vi "StringToNumber.vi"(7 "Conversion type":enum16{"float", "dbl"}(ring), 8 "error in":errorcluster, 10 "String array":string[](array[string]), 11 "String":string) -> (0 "error out":errorcluster, 2 "Number array":dbl[](array[numeric]), 3 "Number":dbl)   [LabVIEW 2019, in "Tools.lvlib"]
uses:
  Tools.lvlib
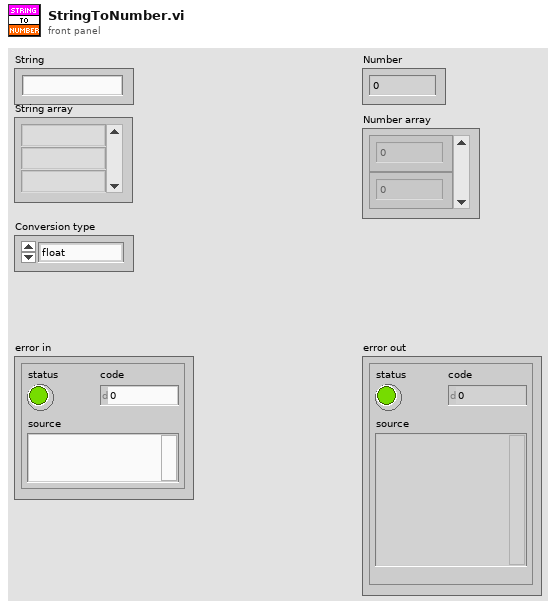
[diagram p1: front panel]
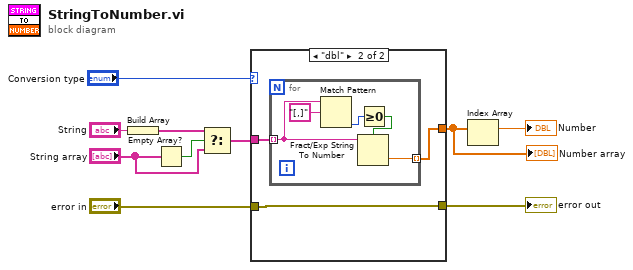
[diagram p0: block diagram]
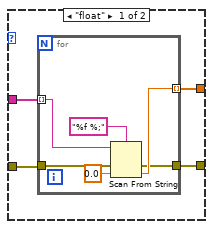
[diagram p2: hidden frame]
diagram:
  n1 = Build Array("String") -> (w4:string[])
  n2 = Empty Array?(array="String array") -> (empty?=w5:bool)
  n3 = Select(t=w4, s=w5, f="String array") -> (s? t:f=w3:string[])
  n4 = case shown="\"dbl\"" "Conversion type" {
    tunnel: [w14 w21] -> w10
    tunnel: [w13 w23] -> w8
    tunnel: "error in" -> [w12 w23]
    tunnel: w3 -> [w11 w22]
    frame "float" {
      n5 = for {
        tunnel: [w20] -> w14 mode=indexing
        tunnel: w11 -> [w19] mode=indexing
        tunnel: w12 -> [w17]
        tunnel: [w18] -> w13
        n6 = Scan From String(format string="%f %;", input string=w19, error in=w17, default 1=0.0 ("default value 1")) -> (error out=w18:errorcluster, output 1=w20:dbl)  [unwired: 1 in, 2 out]
      }
    }
    frame "dbl" {
      n7 = for {
        tunnel: w22 -> [w26] mode=indexing
        tunnel: [w28] -> w21 mode=indexing
        n8 = Match Pattern(string=w26, regular expression="[,]") -> (offset past match=w25:i32)  [unwired: 1 in, 3 out]
        n9 = Greater Or Equal To 0?(x=w25) -> (x >= 0?=w24:bool)
        n10 = Fract/Exp String To Number(use system decimal point (T)=w24, string=w26) -> (number=w28:dbl)  [unwired: 2 in, 1 out]
      }
    }
  }
  "error out" <- w8
  "Number array" <- w10
  n11 = Index Array(array=w10) -> (element=→"Number":dbl)  [unwired: 1 in]
